vi "A_SIG.vi"(0 "LL":dbl, 1 "OutLimMin":dbl, 2 "OutLimMax":dbl, 3 "UL":dbl, 5 "error in (no error)":errorcluster, 8 "Input":dbl) -> (16 "A_SIG_out":dbl, 19 "error out":errorcluster)   [LabVIEW 2022 SP3]
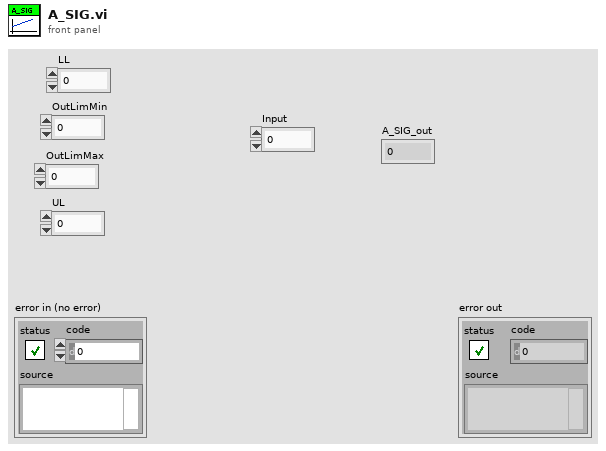
[diagram p1: front panel]
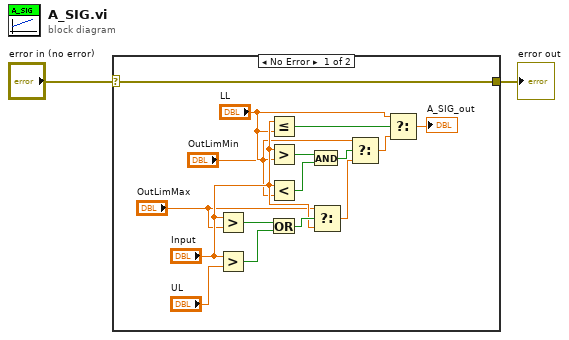
[diagram p0: block diagram]
diagram:
  n1 = case shown="No Error" "error in (no error)" {
    selector: "error in (no error)" -> [w18 w19]
    tunnel: [w18 w19] -> w1
    frame No Error {
      n2 = Greater?(x="Input", y="OutLimMax") -> (0:w13:bool)
      n3 = Greater?(x="Input", y="UL") -> (0:w12:bool)
      n4 = Less Or Equal?(x="Input", y="LL") -> (x <= y?=w17:bool)
      n5 = Greater?(x="Input", y="LL") -> (0:w16:bool)
      n6 = Less?(x="Input", y="OutLimMin") -> (x < y?=w15:bool)
      n7 = Or(x=w13, y=w12) -> (x .or. y?=w11:bool)
      n8 = And(x=w16, y=w15) -> (x .and. y?=w14:bool)
      n9 = Select(t="OutLimMax", s=w11, f="Input") -> (s? t:f=w9:dbl)
      n10 = Select(t="OutLimMin", s=w14, f=w9) -> (s? t:f=w8:dbl)
      n11 = Select(t="LL", s=w17, f=w8) -> (s? t:f=→"A_SIG_out":dbl)
    }
    frame Error {
    }
  }
  "error out" <- w1
